vi "Client LabVIEW.vi"() -> ()   [LabVIEW 2014]
panel:
  in  "Port":u16=5001
  in  "Address":string="172.28.16.1"
  in  "Aturar connexió":bool
  out "Codi d'error":string
  out "Comptador":dbl
  out "Mínim":dbl
  out "Mitjana":dbl
  out "Waveform Chart":dbl(graph)
  out "Màxim":dbl
  in  "Enviar missatge":bool
  in  "Marxa/parada":bool
  in  "Nº mostres":i32
  in  "Temps":i32 format="%02d"
  in  "Escull una acció":u16(ring) items=["Posar en marxa / parar adquisició", "Demanar la mitjana", "Demanar màxim", "Demanar mínim", "Reset màxim/mínim", " Nombre de mostres guardades"]
  out "Missatge del servidor":string
  # "ADREÇA"
  # "PARÀMETRES"
  # "M"
  # "P"
  # "DADES"
  # "RESPOSTA DEL SERVIDOR"
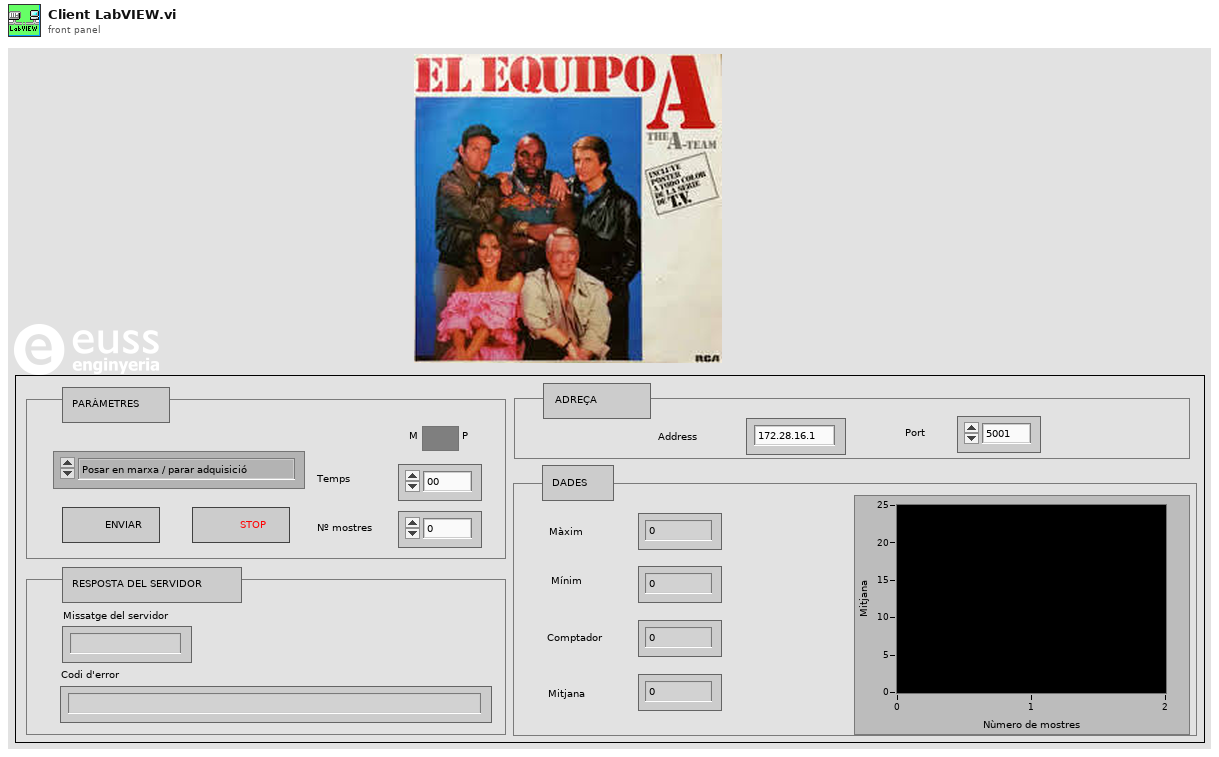
[diagram p1: front panel]
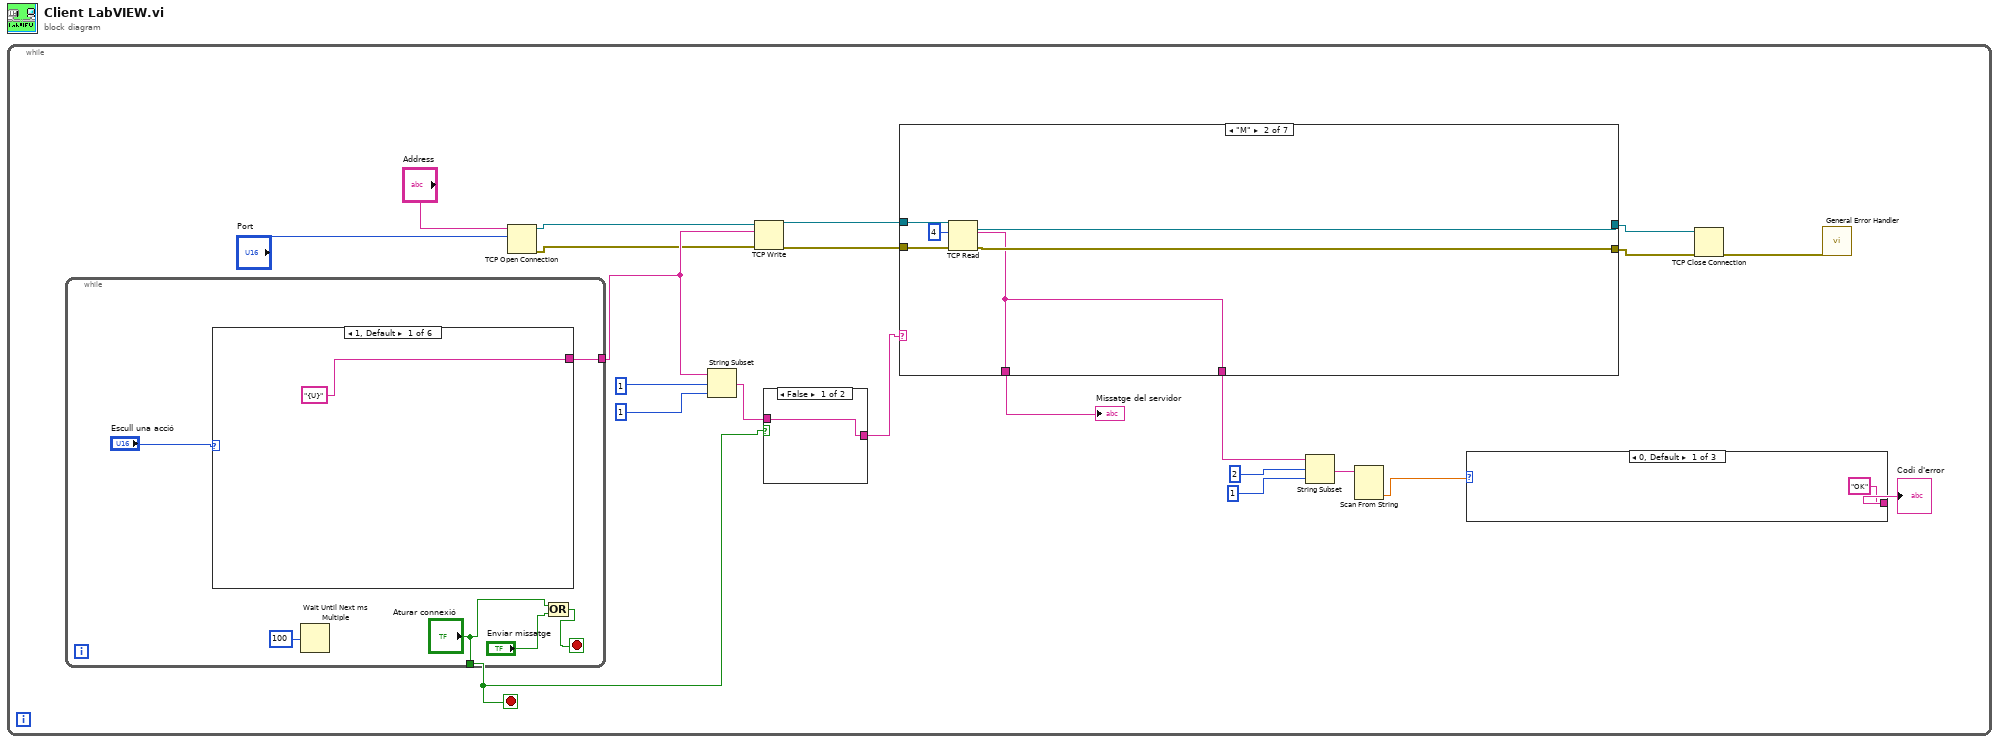
[diagram p0: block diagram]
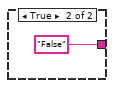
[diagram p2: hidden frame]
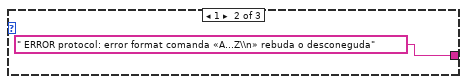
[diagram p3: hidden frame]
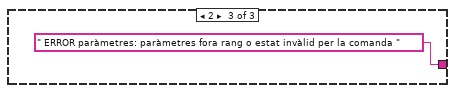
[diagram p4: hidden frame]
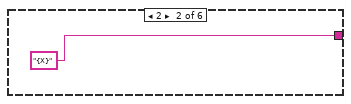
[diagram p5: hidden frame]
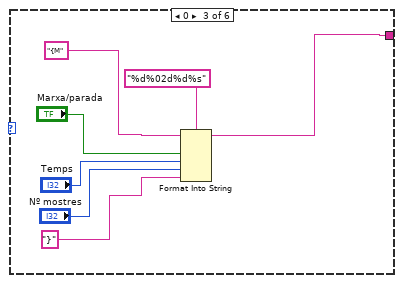
[diagram p6: hidden frame]
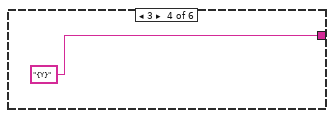
[diagram p7: hidden frame]
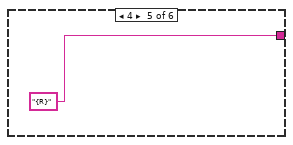
[diagram p8: hidden frame]
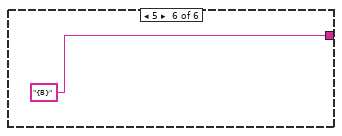
[diagram p9: hidden frame]
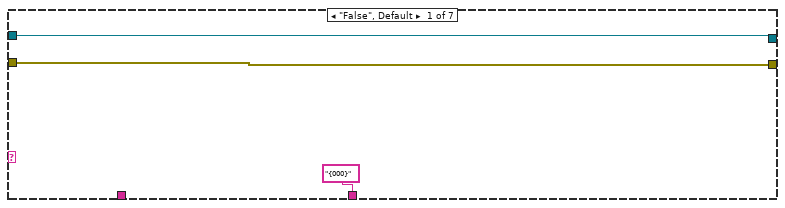
[diagram p10: hidden frame]
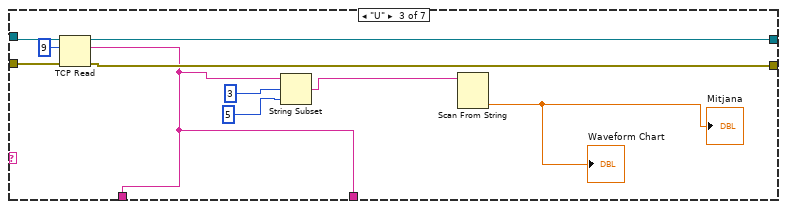
[diagram p11: hidden frame]
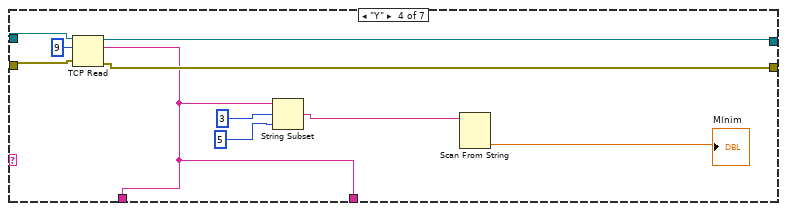
[diagram p12: hidden frame]
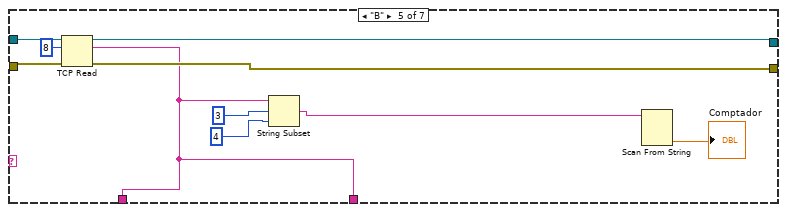
[diagram p13: hidden frame]
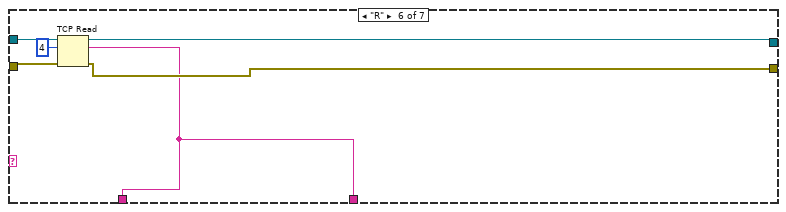
[diagram p14: hidden frame]
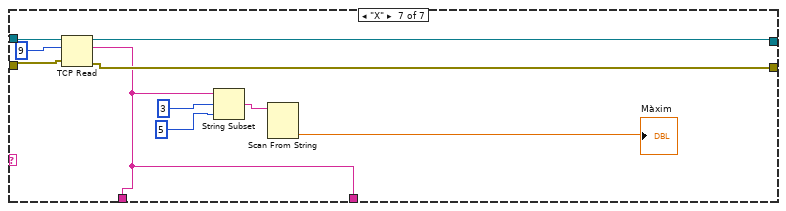
[diagram p15: hidden frame]
diagram:
  n1 = while {
    stop <- w3 stop-if-true
    n2 = while {
      tunnel: [w32] -> w18
      tunnel: ["Aturar connexió"] -> w3
      stop <- w28 stop-if-true
      n3 = case shown="1, Default" "Escull una acció" {
        tunnel: ["{U}" "{X}" w36 "{Y}" "{R}" "{B}"] -> w32
        frame 1, Default {
        }
        frame 2 {
        }
        frame 0 {
          n4 = Format Into String(format string="%d%02d%d%s", initial string="{M", "Marxa/parada", "Temps", "Nº mostres", "}") -> (resulting string=w36:string)  [unwired: 1 in, 1 out]
        }
        frame 3 {
        }
        frame 4 {
        }
        frame 5 {
        }
      }
      n5 = Wait Until Next ms Multiple(millisecond multiple=u32 100) -> ()  [unwired: 1 out]
      n6 = Or(x="Aturar connexió", y="Enviar missatge") -> (x .or. y?=w28:bool)
    }
    n7 = TCP Open Connection(address="Address", remote port or service name="Port") -> (connection ID=w8:refnum<k5>, error out=w7:errorcluster)  [unwired: 3 in]
    n8 = String Subset(string=w18, offset (0)=1, length (rest)=1 ("length (rest)")) -> (substring=w2:string)
    n9 = TCP Write(connection ID=w8, data in=w18, error in (no error)=w7) -> (connection ID out=w20:refnum<k5>, error out=w19:errorcluster)  [unwired: 1 in, 1 out]
    n10 = case shown="False" w3 {
      tunnel: [w23 "False"] -> w1
      tunnel: w2 -> [w23 _]
      frame False {
      }
      frame True {
      }
    }
    n11 = case shown="\"M\"" w1 {
      tunnel: w20 -> [w48 w53 w63 w73 w83 w89 w99]
      tunnel: w19 -> [w47 w52 w62 w72 w82 w88 w98]
      tunnel: [w48 w51 w60 w71 w81 w87 w97] -> w5
      tunnel: [w47 w50 w61 w70 w80 w86 w96] -> w4
      tunnel: [_ w49 w56 w66 w76 w85 w92] -> w17
      tunnel: ["{000}" ("data out") w49 w56 w66 w76 w85 w92] -> w13
      frame "False", Default {
      }
      frame "M" {
        n12 = TCP Read(connection ID=w53, bytes to read=4, error in (no error)=w52) -> (connection ID out=w51:refnum<k5>, data out=w49:string, error out=w50:errorcluster)  [unwired: 2 in]
      }
      frame "U" {
        n13 = TCP Read(connection ID=w63, bytes to read=9, error in (no error)=w62) -> (connection ID out=w60:refnum<k5>, data out=w56:string, error out=w61:errorcluster)  [unwired: 2 in]
        n14 = String Subset(string=w56, offset (0)=3, length (rest)=5 ("offset (0)")) -> (substring=w57:string)
        n15 = Scan From String(input string=w57) -> (output 1=→"Mitjana" →"Waveform Chart":dbl)  [unwired: 4 in, 3 out]
      }
      frame "Y" {
        n16 = TCP Read(connection ID=w73, bytes to read=9, error in (no error)=w72) -> (connection ID out=w71:refnum<k5>, data out=w66:string, error out=w70:errorcluster)  [unwired: 2 in]
        n17 = String Subset(string=w66, offset (0)=3, length (rest)=5 ("offset (0)")) -> (substring=w67:string)
        n18 = Scan From String(input string=w67) -> (output 1=→"Mínim":dbl)  [unwired: 4 in, 3 out]
      }
      frame "B" {
        n19 = TCP Read(connection ID=w83, bytes to read=8, error in (no error)=w82) -> (connection ID out=w81:refnum<k5>, data out=w76:string, error out=w80:errorcluster)  [unwired: 2 in]
        n20 = String Subset(string=w76, offset (0)=3, length (rest)=4 ("offset (0)")) -> (substring=w77:string)
        n21 = Scan From String(input string=w77) -> (output 1=→"Comptador":dbl)  [unwired: 4 in, 3 out]
      }
      frame "R" {
        n22 = TCP Read(connection ID=w89, bytes to read=4, error in (no error)=w88) -> (connection ID out=w87:refnum<k5>, data out=w85:string, error out=w86:errorcluster)  [unwired: 2 in]
      }
      frame "X" {
        n23 = TCP Read(connection ID=w99, bytes to read=9, error in (no error)=w98) -> (connection ID out=w97:refnum<k5>, data out=w92:string, error out=w96:errorcluster)  [unwired: 2 in]
        n24 = String Subset(string=w92, offset (0)=3, length (rest)=5 ("offset (0)")) -> (substring=w93:string)
        n25 = Scan From String(input string=w93) -> (output 1=→"Màxim":dbl)  [unwired: 4 in, 3 out]
      }
    }
    "Missatge del servidor" <- w17
    n26 = String Subset(string=w13, offset (0)=2, length (rest)=1 ("offset (0)")) -> (substring=w14:string)
    n27 = Scan From String(input string=w14) -> (output 1=w11:dbl)  [unwired: 4 in, 3 out]
    n28 = case shown="0, Default" w11 {
      tunnel: ["OK" ("ERROR") " ERROR protocol: error format comanda «A...Z\\n» rebuda o desconeguda" ("ERROR") " ERROR paràmetres: paràmetres fora rang o estat invàlid per la comanda " ("ERROR")] -> w12
      frame 0, Default {
      }
      frame 1 {
      }
      frame 2 {
      }
    }
    "Codi d'error" <- w12
    n29 = TCP Close Connection(connection ID=w5, error in (no error)=w4) -> (error out=w6:errorcluster)  [unwired: 1 in, 1 out]
    n30 = call <vilib>:"General Error Handler.vi"("error in (no error)"=w6) -> ()  [unwired: 10 in, 5 out]
  }
